vi "Tree_Setup for dialog.vi"(7 "Action":T1, 8 "error in":errorcluster, 11 "Tree Ref":refnum<vi>[](array[refnum])) -> (0 "error out":errorcluster, 3 "Tree Ref Out":refnum<vi>[](array[refnum]))   [LabVIEW 2023]
doc: "This VI sets up tree-level, but NOT row-level settings."
uses:
  controls/action enum.ctl
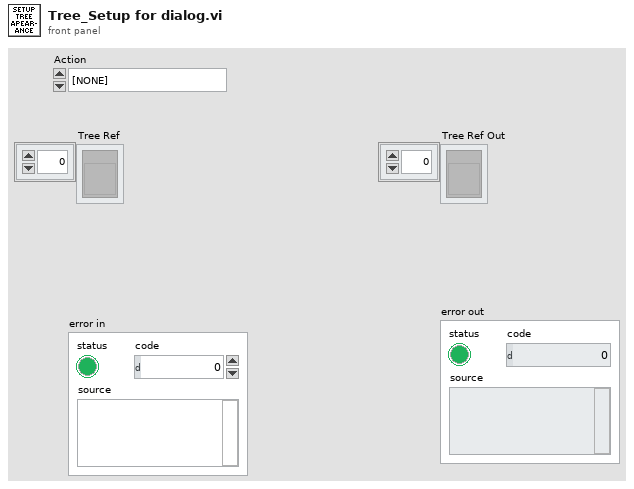
[diagram p1: front panel]
types:
  T1 = typedef "action enum.ctl" = enum16{"[NONE]", "Wire Bundle", "Wire Unbundle", "Terminal Unbundle", "Terminal Bundle", "Bundler Move Up", "Bundler Move Down", "Bundler Insert", "Bundler Remove", "Bundler Remove Unwired", "Bundler Rearrange", "In Place Insert", "In Place Remove", "In Place Remove Unwired", "In Place Rearrange", "Wire Properties", "Wire Method", "Terminal Properties", "Terminal Method", "Property Move Up", "Property Move Down", "Properties Insert", "Properties Remove", "Properties Remove Unwired", "Properties Rearrange", "Method Change", "Class for Constant", "Class For Control", "Class For Node", "Class Name to Clipboard"}
  T2 = enum16{"[NONE]", "Wire Bundle", "Wire Unbundle", "Terminal Unbundle", "Terminal Bundle", "Bundler Insert", "Bundler Remove", "Bundler Remove Unwired", "Bundler Rearrange", "In Place Insert", "In Place Remove", "In Place Remove Unwired", "In Place Rearrange", "Wire Properties", "Wire Method", "Terminal Properties", "Terminal Method", "Properties Insert", "Properties Remove", "Properties Remove Unwired", "Properties Rearrange", "Method Change", "Class for Constant", "Class For Control", "Class For Node", "Class Name to Clipboard"}
  T3 = enum32{"None", "LabVIEW", "Mac OS", "Windows", "Default"}
  T4 = enum8{"Enabled", "Disabled", "Disabled and Grayed Out"}
  T5 = enum16{"None", "Cluster", "Property", "Method", "Class"}
  T6 = cluster{"image type":i32, "image depth":i32, "image":u8[], "mask":u8[], "colors":u32[], "Rectangle":cluster{"left":i16, "top":i16, "right":i16, "bottom":i16}}
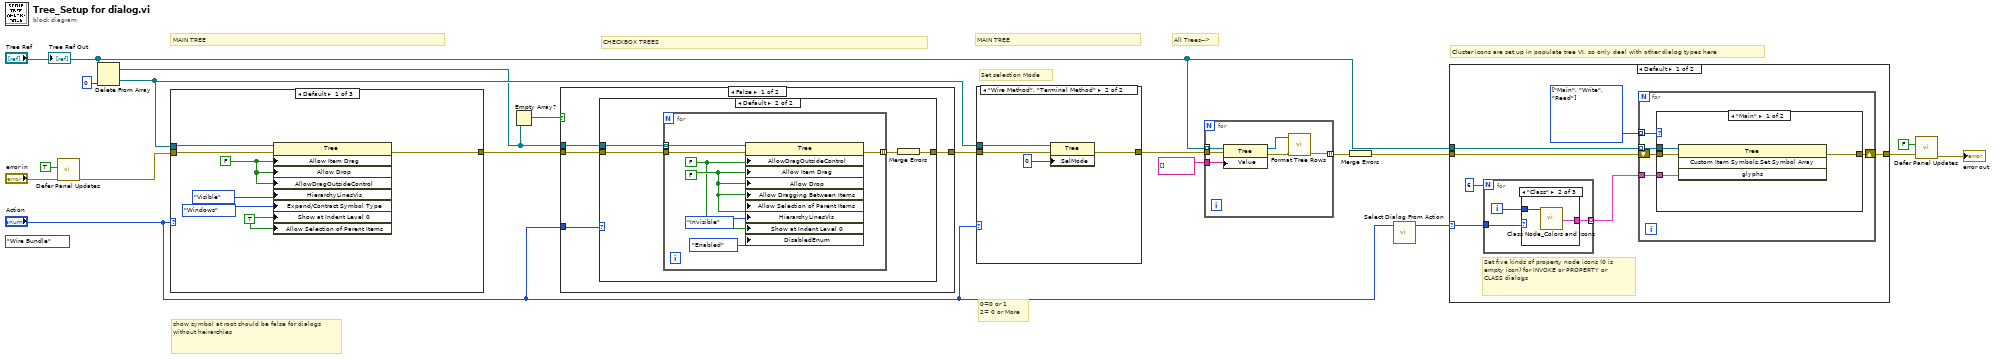
[diagram p0: block diagram]
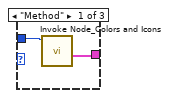
[diagram p2: hidden frame]
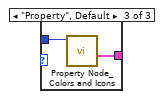
[diagram p3: hidden frame]
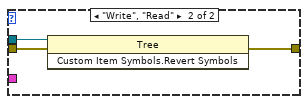
[diagram p4: hidden frame]
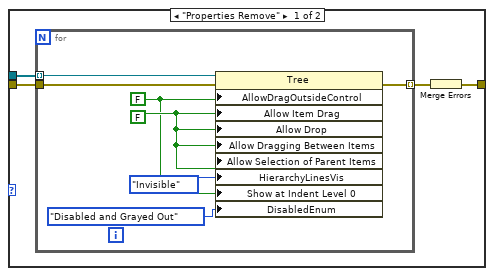
[diagram p6: hidden frame]
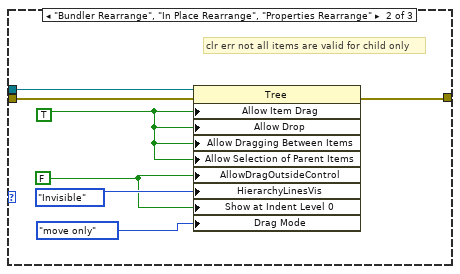
[diagram p8: hidden frame]
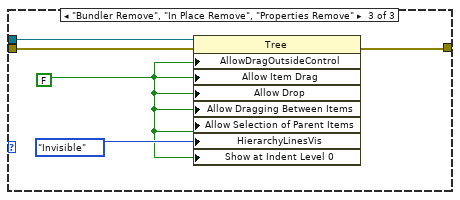
[diagram p9: hidden frame]
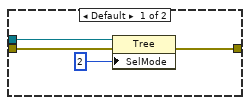
[diagram p10: hidden frame]
diagram:
  (unwired) T2."Wire Bundle" ("Action")
  # "Cluster icons are set up in populate tree VI, so only deal with other dialog types here"
  # "All Trees-->"
  # "MAIN TREE"
  # "show symbol at root should be false for dialogs without heirarchies"
  # "CHECKBOX TREES"
  # "MAIN TREE"
  # "Set selection Mode"
  # "0=0 or 1\n2= 0 or More"
  n1 = call "Defer Panel Updates.vi"("error in (no error)"="error in", "Defer Panel Updates [T]"=TRUE) -> ("error out"=w10:errorcluster)  [unwired: 8 in, 1 out]
  n2 = Delete From Array(array="Tree Ref", index=0) -> (deleted portion=w6:refnum<vi>, array with subset deleted=w3:refnum<vi>[])  [unwired: 1 in]
  n3 = case shown="Default" "Action" {
    tunnel: w6 -> [w26 w33 w38]
    tunnel: [w24 w27 w36] -> w8
    tunnel: w10 -> [w25 w32 w37]
    frame Default {
      w22 = TRUE
      w21 = FALSE
      n4 = property class="Tree"(reference=w26, error in=w25, "Allow Item Drag"=w21, "Allow Drop"=w21, "AllowDragOutsideControl"=w21, "HierarchyLinesVis"=enum32{"Visible", "Invisible", "OS Default"}."Visible" ("Visible Items:Hierarchy Lines Visible"), "Expand/Contract Symbol Type"=T3."Windows" ("Expand/Contract Symbol:Symbol Type"), "Show at Indent Level 0"=w22, "Allow Selection of Parent Items"=w22) -> (error out=w24:errorcluster)  [unwired: 1 out]
    }
    frame "Bundler Rearrange", "In Place Rearrange", "Properties Rearrange" {
      w28 = TRUE
      w29 = FALSE
      # "clr err not all items are valid for child only"
      n5 = property class="Tree"(reference=w33, error in=w32, "Allow Item Drag"=w28, "Allow Drop"=w28, "Allow Dragging Between Items"=w28, "Allow Selection of Parent Items"=w28, "AllowDragOutsideControl"=w29, "HierarchyLinesVis"=enum32{"Visible", "Invisible", "OS Default"}."Invisible" ("Visible Items:Hierarchy Lines Visible"), "Show at Indent Level 0"=w29, "Drag Mode"=enum32{"copy or move", "copy only", "move only"}."move only" ("Drag/Drop:Drag Mode")) -> (error out=w27:errorcluster)  [unwired: 1 out]
    }
    frame "Bundler Remove", "In Place Remove", "Properties Remove" {
      w34 = FALSE
      n6 = property class="Tree"(reference=w38, error in=w37, "AllowDragOutsideControl"=w34, "Allow Item Drag"=w34, "Allow Drop"=w34, "Allow Dragging Between Items"=w34, "Allow Selection of Parent Items"=w34, "HierarchyLinesVis"=enum32{"Visible", "Invisible", "OS Default"}."Invisible" ("Visible Items:Hierarchy Lines Visible"), "Show at Indent Level 0"=w34) -> (error out=w36:errorcluster)  [unwired: 1 out]
    }
  }
  n7 = Empty Array?(array=w3) -> (empty?=w4:bool)
  n8 = case shown="False" w4 {
    tunnel: w3 -> [w42 _]
    tunnel: w8 -> [w41 w65]
    tunnel: [w40 w65] -> w7
    tunnel: "Action" -> [w39 _]
    frame False {
      n9 = case shown="Default" w39 {
        tunnel: w42 -> [w46 w57]
        tunnel: w41 -> [w45 w56]
        tunnel: [w43 w54] -> w40
        frame "Properties Remove" {
          n10 = for {
            tunnel: w46 -> [w53] mode=indexing
            tunnel: w45 -> [w52]
            tunnel: [w51] -> w44 mode=indexing
            w49 = FALSE
            w48 = FALSE
            n11 = property class="Tree"(reference=w53, error in=w52, "AllowDragOutsideControl"=w48, "Allow Item Drag"=w49, "Allow Drop"=w49, "Allow Dragging Between Items"=w49, "Allow Selection of Parent Items"=w49, "HierarchyLinesVis"=enum32{"Visible", "Invisible", "OS Default"}."Invisible" ("Visible Items:Hierarchy Lines Visible"), "Show at Indent Level 0"=w48, "DisabledEnum"=T4."Disabled and Grayed Out" ("Disabled")) -> (error out=w51:errorcluster)  [unwired: 1 out]
          }
          n12 = Merge Errors(w44) -> (w43:errorcluster)
        }
        frame Default {
          n13 = for {
            tunnel: w57 -> [w64] mode=indexing
            tunnel: w56 -> [w63]
            tunnel: [w62] -> w55 mode=indexing
            w60 = FALSE
            w59 = FALSE
            n14 = property class="Tree"(reference=w64, error in=w63, "AllowDragOutsideControl"=w59, "Allow Item Drag"=w60, "Allow Drop"=w60, "Allow Dragging Between Items"=w60, "Allow Selection of Parent Items"=w60, "HierarchyLinesVis"=enum32{"Visible", "Invisible", "OS Default"}."Invisible" ("Visible Items:Hierarchy Lines Visible"), "Show at Indent Level 0"=w59, "DisabledEnum"=T4."Enabled" ("Disabled")) -> (error out=w62:errorcluster)  [unwired: 1 out]
          }
          n15 = Merge Errors(w55) -> (w54:errorcluster)
        }
      }
    }
    frame True {
    }
  }
  n16 = case shown="\"Wire Method\", \"Terminal Method\"" "Action" {
    tunnel: w6 -> [w68 w72]
    tunnel: w7 -> [w67 w71]
    tunnel: [w66 w70] -> w19
    frame Default {
      n17 = property class="Tree"(reference=w68, error in=w67, "SelMode"=2 ("Selection Mode")) -> (error out=w66:errorcluster)  [unwired: 1 out]
    }
    frame "Wire Method", "Terminal Method" {
      n18 = property class="Tree"(reference=w72, error in=w71, "SelMode"=0 ("Selection Mode")) -> (error out=w70:errorcluster)  [unwired: 1 out]
    }
  }
  n19 = for {
    tunnel: "Tree Ref" -> [w79] mode=indexing
    tunnel: w19 -> [w78]
    tunnel: [w74] -> w18 mode=indexing
    tunnel: string[] [] ("Value") -> [w77]
    n20 = property class="Tree"(reference=w79, error in=w78, "Value"=w77) -> (reference out=w75:refnum<vi>, error out=w76:errorcluster)
    n21 = call "Format Tree Rows.vi"("error in"=w76, "Tree Ref"=w75) -> ("error out"=w74:errorcluster)  [unwired: 8 in, 1 out]
  }
  n22 = Merge Errors(w18) -> (w17:errorcluster)
  n23 = call "Select Dialog From Action.vi"("Action"="Action") -> ("Dialog Selection"=w1:T5)  [unwired: 10 in]
  n24 = case shown="Default" w1 {
    selector: w1 -> [w80 _]
    tunnel: w17 -> [w86 w108]
    tunnel: [w85 w108] -> w13
    tunnel: "Tree Ref" -> [w84 _]
    frame Default {
      w81 = enum16{"Main", "Write", "Read"}[] [enum."Main", enum."Write", enum."Read"] items=["Main", "Write", "Read"] ("Tree Type")
      # "Set five kinds of property node icons (0 is empty icon) for INVOKE or PROPERTY or CLASS dialogs"
      n25 = for {
        N: 6 -> [_]
        tunnel: [w88] -> w83 mode=indexing
        tunnel: w80 -> [w87]
        i -> [w89]
        n26 = case shown="\"Class\"" w87 {
          tunnel: w89 -> [w91 w93 w95]
          tunnel: [w90 w92 w94] -> w88
          frame "Method" {
            n27 = call "Invoke Node_Colors and Icons.vi"("Property Type"=w91) -> ("Icon Pixmap"=w90:T6)  [unwired: 8 in, 2 out]
          }
          frame "Class" {
            n28 = call "Class Node_Colors and Icons.vi"("Property Type"=w93) -> ("Icon Pixmap"=w92:T6)  [unwired: 8 in, 2 out]
          }
          frame "Property", Default {
            n29 = call "Property Node_Colors and Icons.vi"("Property Type"=w95) -> ("Icon Pixmap"=w94:T6)  [unwired: 8 in, 2 out]
          }
        }
      }
      n30 = for {
        tunnel: w83 -> [w100]
        tunnel: w84 -> [w99] mode=indexing
        shift-right: [w97] -> w85
        shift-left: w86 -> [w98]
        tunnel: w81 -> [w96] mode=indexing
        n31 = case shown="\"Main\"" w96 {
          tunnel: [w101 w105] -> w97
          tunnel: w99 -> [w104 w107]
          tunnel: w98 -> [w103 w106]
          tunnel: w100 -> [w102 _]
          frame "Main" {
            n32 = invoke class="Tree" method="Custom Item Symbols.Set Symbol Array"(reference=w104, error in=w103, "glyphs"=w102) -> (error out=w101:errorcluster)  [unwired: 1 in, 3 out]
          }
          frame "Write", "Read" {
            n33 = invoke class="Tree" method="Custom Item Symbols.Revert Symbols"(reference=w107, error in=w106) -> (error out=w105:errorcluster)  [unwired: 1 in, 2 out]
          }
        }
      }
    }
    frame "Cluster" {
    }
  }
  n34 = call "Defer Panel Updates.vi"("error in (no error)"=w13, "Defer Panel Updates [T]"=FALSE) -> ("error out"=→"error out":errorcluster)  [unwired: 8 in, 1 out]
  "Tree Ref Out" <- "Tree Ref"
